vi "SetClassWireColor.vi"(8 "error in (no error)":errorcluster, 10 "Color":u32(colorbox), 11 "LVClassLibrary Refnum":refnum<vi>) -> (0 "error out":errorcluster, 3 "Library Refnum out":refnum<vi>)   [LabVIEW 2014, in "ClassIconTools.lvlib"]
uses:
  ClassIconTools.lvlib
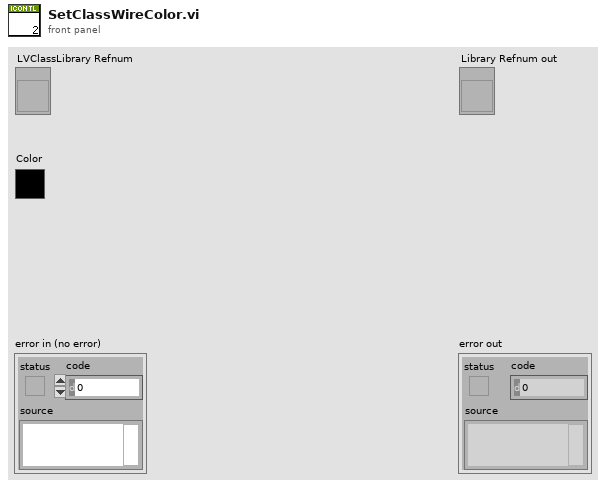
[diagram p1: front panel]
types:
  T1 = cluster{"Foreground Color":u32, "Background Color":u32, "Fill Pattern":cluster{"Row 0":u8, "Row 1":u8, "Row 2":u8, "Row 3":u8, "Row 4":u8, "Row 5":u8, "Row 6":u8, "Row 7":u8}, "Width":i16, "Mode":enum16{"Copy", "Or", "Exclusive Or", "Bit Clear", "Not Copy", "Not Or", "Nor Exclusive Or", "Not Bit Clear"}, "Style":enum32{"Solid", "Dash", "Dot", "Dash Dot", "Dash Dot Dot"}, "Fill Rule":enum32{"Even Odd", "Winding"}, "End Caps":enum32{"Default", "Flat"}}[]
  T2 = cluster{"Foreground Color":u32, "Background Color":u32, "Fill Pattern":cluster{"Row 0":u8, "Row 1":u8, "Row 2":u8, "Row 3":u8, "Row 4":u8, "Row 5":u8, "Row 6":u8, "Row 7":u8}, "Width":i16, "Mode":enum16{"Copy", "Or", "Exclusive Or", "Bit Clear", "Not Copy", "Not Or", "Nor Exclusive Or", "Not Bit Clear"}, "Style":enum32{"Solid", "Dash", "Dot", "Dash Dot", "Dash Dot Dot"}, "Fill Rule":enum32{"Even Odd", "Winding"}, "End Caps":enum32{"Default", "Flat"}}
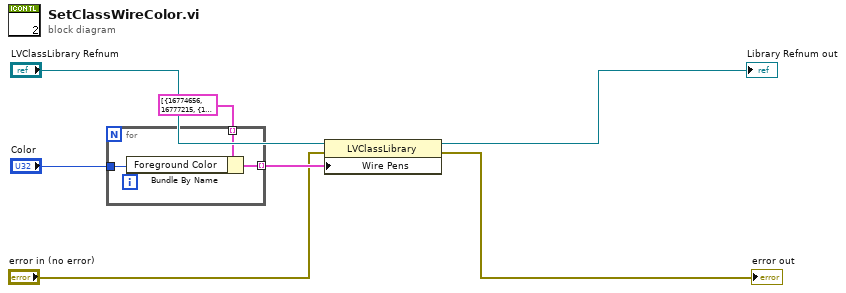
[diagram p0: block diagram]
diagram:
  n1 = for {
    tunnel: T1 [{"Foreground Color"=16774656, "Background Color"=16777215, "Fill Pattern"={"Row 0"=195, "Row 1"=195, "Row 2"=195, "Row 3"=195, "Row 4"=195, "Row 5"=195, "Row 6"=195, "Row 7"=195}, "Width"=1, "Mode"=enum."Copy", "Style"=enum."Solid", "Fill Rule"=enum."Even Odd", "End Caps"=enum."Default"}, {"Foreground Color"=12845153, "Background Color"=16777215, "Fill Pattern"={"Row 0"=126, "Row 1"=126, "Row 2"=126, "Row 3"=126, "Row 4"=126, "Row 5"=126, "Row 6"=126, "Row 7"=126}, "Width"=3, "Mode"=enum."Copy", "Style"=enum."Solid", "Fill Rule"=enum."Even Odd", "End Caps"=enum."Default"}] ("Wire Pens") -> [w10] mode=indexing
    tunnel: [w9] -> w5 mode=indexing
    tunnel: "Color" -> [w8]
    n2 = Bundle By Name(cluster=w10, "Foreground Color"=w8) -> (w9:T2)
  }
  n3 = property class="LVClassLibrary"(reference="LVClassLibrary Refnum", error in="error in (no error)", "Wire Pens"=w5) -> (reference out=→"Library Refnum out":refnum<vi>, error out=→"error out":errorcluster)
